vi "GOMDBTS2048 calib Measure Integral.vi"(8 "error in (no error)":errorcluster, 11 "handle":i32) -> (0 "error out":errorcluster, 1 "calFactor":dbl, 2 "currentSignal":dbl, 3 "currentDark":dbl, 5 "function return":i32)   [LabVIEW 2015, in "GOMDBTS2048.lvlib"]
doc: "GOBTS2048DLL int __stdcall GOMDBTS2048_calibMeasureIntegral(int handle, double* currentDark, double* currentSignal, double* calFactor);"
uses:
  GOMDBTS2048.lvlib
  runtime/GOMDBTS2048.dll
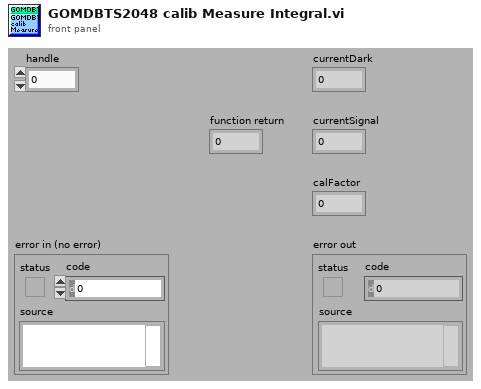
[diagram p1: front panel]
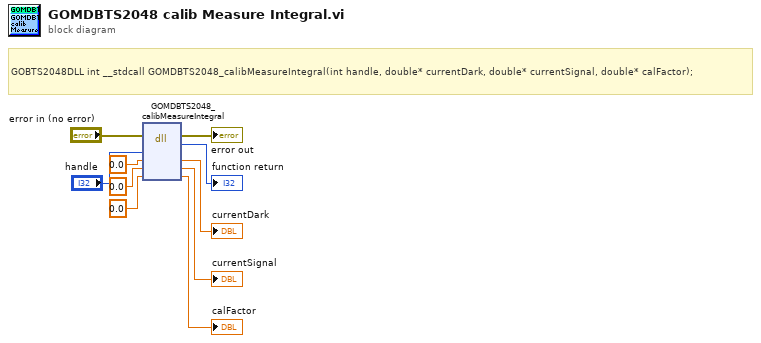
[diagram p0: block diagram]
diagram:
  # "GOBTS2048DLL int __stdcall GOMDBTS2048_calibMeasureIntegral(int handle, double* currentDark, double* currentSignal, double* calFactor);"
  n1 = dll-call lib="C:/Users/rkoch/Documents/GO_Library/runtime/GOMDBTS2048.*" fn="GOMDBTS2048_calibMeasureIntegral"(error in="error in (no error)", "handle"="handle", "currentDark"=0.0, "currentSignal"=0.0, "calFactor"=0.0) -> (error out=→"error out":errorcluster, →"function return":i32, "currentDark"=→"currentDark":dbl, "currentSignal"=→"currentSignal":dbl, "calFactor"=→"calFactor":dbl)  [unwired: 3 in, 1 out]
